vi "ReadInfo.vi"(7 "error in (no error)":errorcluster, 9 "XPath expression":string="/COOLER_STATUS/LIST_OF_INFO/INFO", 10 "path to XML document in":path caption="path to XML") -> (0 "error out":errorcluster, 1 "value":string[](array[string]), 2 "Info":string[](array[string]), 3 "path to XML document out":path caption="path to XML")   [LabVIEW 2017]
uses:
  <vilib>/xml/Load XML File.vi
  <vilib>/xml/Close Reference(Node).vi
  <resource>/objmgr/DOMUserDefRef.rc
  <vilib>/xml/NI_XML.lvlib
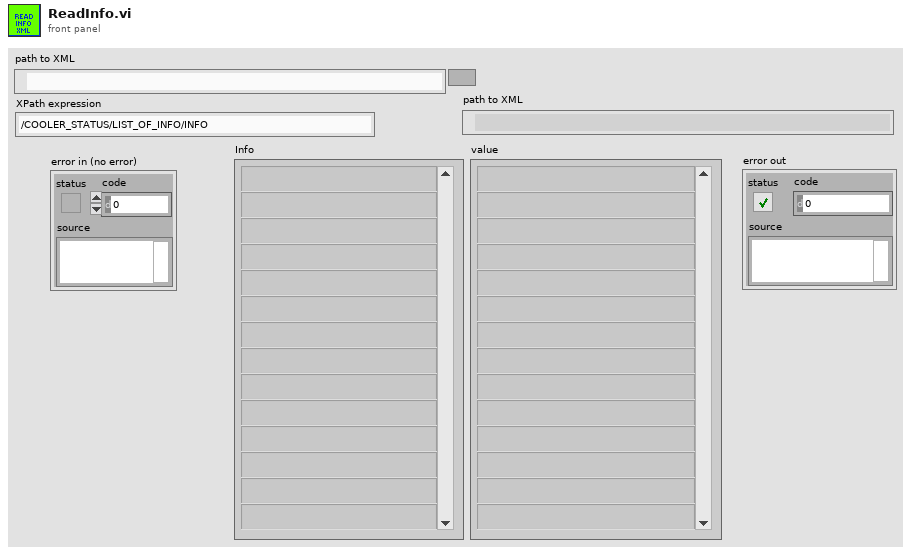
[diagram p1: front panel]
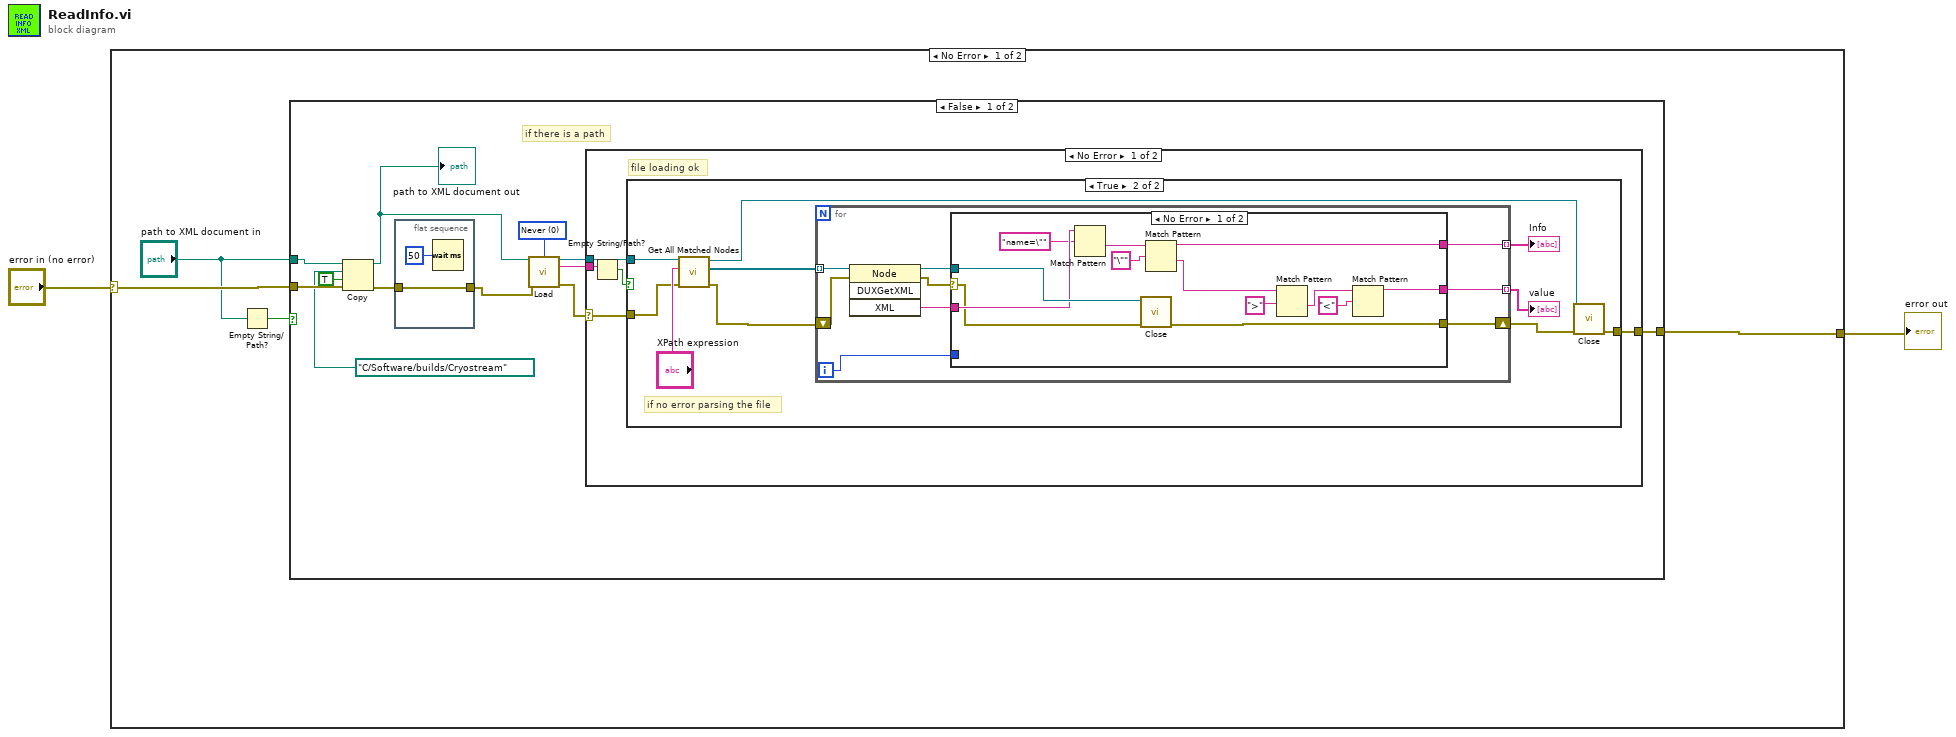
[diagram p0: block diagram]
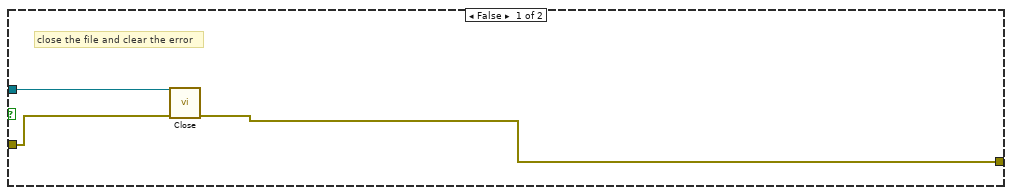
[diagram p2: hidden frame]
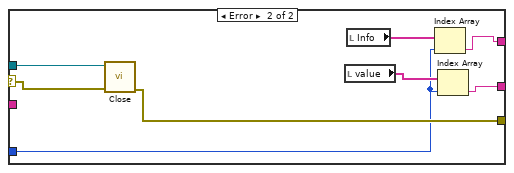
[diagram p3: hidden frame]
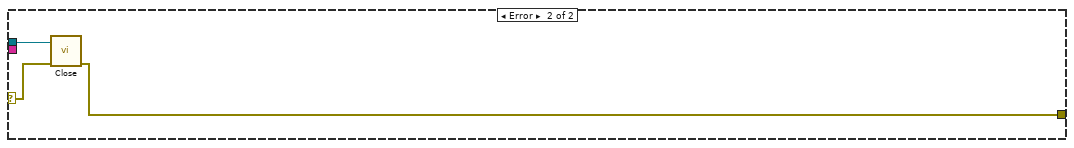
[diagram p4: hidden frame]
diagram:
  n1 = case shown="No Error" "error in (no error)" {
    selector: "error in (no error)" -> [w4 w73]
    tunnel: [w5 w73] -> w2
    frame No Error {
      n2 = Empty String/Path?(string/path="path to XML document in") -> (empty?=w6:bool)
      n3 = case shown="False" w6 {
        tunnel: "path to XML document in" -> [w10 _]
        tunnel: w4 -> [w13 w72]
        tunnel: [w17 w72] -> w5
        frame False {
          w14 = 0 items=["Never", "Always", "Auto"] ("validate on load (Auto)")
          # "if there is a path"
          n4 = Copy(8:w13, 9:TRUE ("overwrite (F)"), 10:path "C:/Software/builds/Cryostream" ("target path (use dialog)"), 11:w10) -> (0:w12:errorcluster, 3:w7:path)  [unwired: 1 in, 1 out]
          "path to XML document out" <- w7
          n5 = flat-sequence {
            tunnel: w12 -> [w19]
            tunnel: [w19] -> w11
            frame #0 {
              n6 = Wait (ms)(milliseconds to wait=u32 50) -> ()  [unwired: 1 out]
            }
          }
          n7 = call-poly <vilib>:"Load.vi"("path to XML document"=w7, "validate on load (Auto)"=w14, "error in (no error)"=w11) -> ("DOM document out"=w18:refnum<k20>, "parse errors"=w16:string, "error out"=w15:errorcluster)  [unwired: 10 in]
          n8 = case shown="No Error" w15 {
            selector: w15 -> [w21 w70]
            tunnel: w18 -> [w25 w71]
            tunnel: [w24 w69] -> w17
            tunnel: w16 -> [w23 _]
            frame No Error {
              # "file loading ok"
              n9 = Empty String/Path?(string/path=w23) -> (empty?=w22:bool)
              n10 = case shown="True" w22 {
                tunnel: w25 -> [w28 w37]
                tunnel: [w27 w33] -> w24
                tunnel: w21 -> [w26 w29]
                frame False {
                  # "close the file and clear the error"
                  n11 = call-poly <vilib>:"Close.vi"("error in (no error)"=w26, "node"=w28) -> ("error out"=w27:errorcluster)  [unwired: 7 in]
                }
                frame True {
                  # "if no error parsing the file"
                  n12 = call <vilib>:"Get All Matched Nodes.vi"("error in (no error)"=w29, "XPath expression"="XPath expression", "node in"=w37) -> ("error out"=w30:errorcluster, "node result array"=w38:refnum<k20>[], "node out"=w32:refnum<k20>)  [unwired: 6 out]
                  n13 = for {
                    tunnel: w38 -> [w46] mode=indexing
                    tunnel: [w43] -> w35 mode=indexing
                    tunnel: [w44] -> w36 mode=indexing
                    shift-right: [w42] -> w31
                    shift-left: w30 -> [w41]
                    i -> [w39]
                    n14 = invoke on="Invoke Node" class="Node" method="DUXGetXML"(reference=w46, error in=w41) -> (reference out=w47:refnum<k20>, error out=w40:errorcluster, "XML"=w45:string)  [unwired: 2 in, 1 out]
                    n15 = case shown="No Error" w40 {
                      selector: w40 -> [w48 w61]
                      tunnel: w47 -> [w60 w68]
                      tunnel: w45 -> [w59 _]
                      tunnel: [w52 w62] -> w44
                      tunnel: [w50 w63] -> w43
                      tunnel: [w49 w67] -> w42
                      tunnel: w39 -> [_ w64]
                      frame No Error {
                        n16 = Match Pattern(string=w59, regular expression="name=\"") -> (after substring=w57:string)  [unwired: 1 in, 3 out]
                        n17 = call-poly <vilib>:"Close.vi"("error in (no error)"=w48, "node"=w60) -> ("error out"=w49:errorcluster)  [unwired: 7 out]
                        n18 = Match Pattern(string=w57, regular expression="\"") -> (before substring=w50:string, after substring=w51:string)  [unwired: 1 in, 2 out]
                        n19 = Match Pattern(string=w51, regular expression=">") -> (after substring=w54:string)  [unwired: 1 in, 3 out]
                        n20 = Match Pattern(string=w54, regular expression="<") -> (before substring=w52:string)  [unwired: 1 in, 3 out]
                      }
                      frame Error {
                        n21 = call-poly <vilib>:"Close.vi"("error in (no error)"=w61, "node"=w68) -> ("error out"=w67:errorcluster)  [unwired: 7 out]
                        n22 = local read "value"() -> (w65:string[])
                        n23 = local read "Info"() -> (w66:string[])
                        n24 = Index Array(array=w66, index=w64) -> (element=w63:string)
                        n25 = Index Array(array=w65, index=w64) -> (element=w62:string)
                      }
                    }
                  }
                  "Info" <- w35
                  "value" <- w36
                  n26 = call-poly <vilib>:"Close.vi"("error in (no error)"=w31, "node"=w32) -> ("error out"=w33:errorcluster)  [unwired: 7 out]
                }
              }
            }
            frame Error {
              n27 = call-poly <vilib>:"Close.vi"("error in (no error)"=w70, "node"=w71) -> ("error out"=w69:errorcluster)  [unwired: 7 in]
            }
          }
        }
        frame True {
        }
      }
    }
    frame Error {
    }
  }
  "error out" <- w2
